vi "HEWH RLT Release Notifier References.vi"(8 "error in (no error)":errorcluster) -> (0 "error out":errorcluster)   [LabVIEW 2020]
uses:
  Type Definitions/HEWH Power Elements.ctl
  Utility/Type Definitions/UTILITY Notifier.ctl
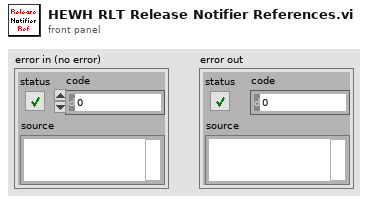
[diagram p1: front panel]
types:
  T1 = typedef "UTILITY Notifier.ctl" = enum16{"Set", "Read", "Release Ref"}
  T2 = typedef "HEWH Power Elements.ctl" = cluster{"UE":bool, "LE":bool, "COMP":bool, "FANS":bool}
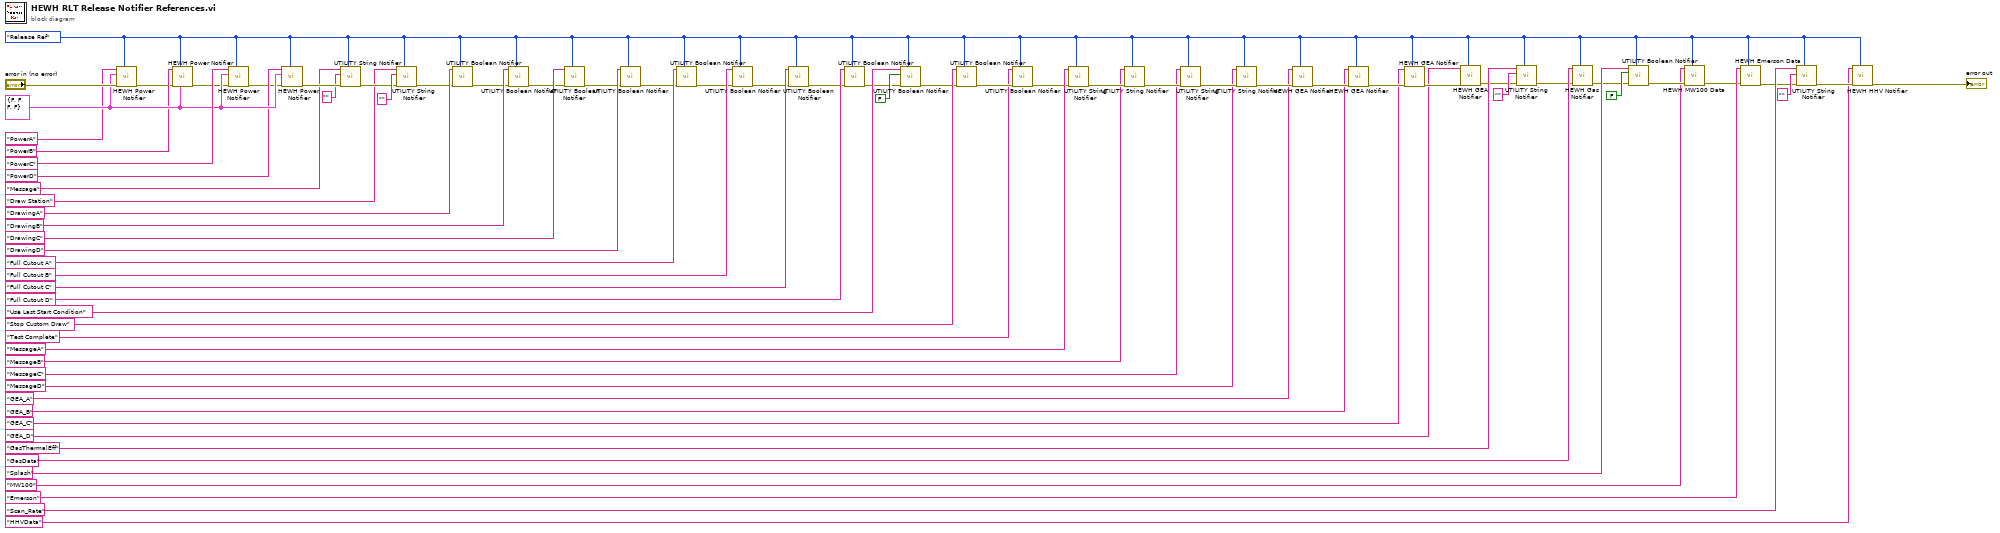
[diagram p0: block diagram]
diagram:
  w2 = UTILITY_Notifier."Release Ref" ("Status")
  w64 = T2 {"UE"=FALSE, "LE"=FALSE, "COMP"=FALSE, "FANS"=FALSE} ("Power Elements")
  n1 = call "HEWH Power Notifier.vi"("Status"=w2, "error in (no error)"="error in (no error)", "Set Status"=w64, "name (unnamed)"="PowerA") -> ("error out"=w59:errorcluster)  [unwired: 6 in, 1 out]
  n2 = call "HEWH Power Notifier.vi"("Status"=w2, "error in (no error)"=w59, "Set Status"=w64, "name (unnamed)"="PowerB") -> ("error out"=w61:errorcluster)  [unwired: 6 in, 1 out]
  n3 = call "HEWH Power Notifier.vi"("Status"=w2, "error in (no error)"=w61, "Set Status"=w64, "name (unnamed)"="PowerC") -> ("error out"=w62:errorcluster)  [unwired: 6 in, 1 out]
  n4 = call "HEWH Power Notifier.vi"("Status"=w2, "error in (no error)"=w62, "Set Status"=w64, "name (unnamed)"="PowerD") -> ("error out"=w69:errorcluster)  [unwired: 6 in, 1 out]
  n5 = call "UTILITY String Notifier.vi"("Status"=w2, "error in (no error)"=w69, "Set Status"="", "name (unnamed)"="Message") -> ("error out"=w71:errorcluster)  [unwired: 6 in, 1 out]
  n6 = call "UTILITY String Notifier.vi"("Status"=w2, "error in (no error)"=w71, "Set Status"="", "name (unnamed)"="Draw Station") -> ("error out"=w53:errorcluster)  [unwired: 6 in, 1 out]
  n7 = call "UTILITY Boolean Notifier.vi"("Status"=w2, "error in (no error)"=w53, "name (unnamed)"="DrawingA") -> ("error out"=w52:errorcluster)  [unwired: 7 in, 1 out]
  n8 = call "UTILITY Boolean Notifier.vi"("Status"=w2, "error in (no error)"=w52, "name (unnamed)"="DrawingB") -> ("error out"=w51:errorcluster)  [unwired: 7 in, 1 out]
  n9 = call "UTILITY Boolean Notifier.vi"("Status"=w2, "error in (no error)"=w51, "name (unnamed)"="DrawingC") -> ("error out"=w50:errorcluster)  [unwired: 7 in, 1 out]
  n10 = call "UTILITY Boolean Notifier.vi"("Status"=w2, "error in (no error)"=w50, "name (unnamed)"="DrawingD") -> ("error out"=w45:errorcluster)  [unwired: 7 in, 1 out]
  n11 = call "UTILITY Boolean Notifier.vi"("Status"=w2, "error in (no error)"=w45, "name (unnamed)"="Full Cutout A") -> ("error out"=w44:errorcluster)  [unwired: 7 in, 1 out]
  n12 = call "UTILITY Boolean Notifier.vi"("Status"=w2, "error in (no error)"=w44, "name (unnamed)"="Full Cutout B") -> ("error out"=w43:errorcluster)  [unwired: 7 in, 1 out]
  n13 = call "UTILITY Boolean Notifier.vi"("Status"=w2, "error in (no error)"=w43, "name (unnamed)"="Full Cutout C") -> ("error out"=w42:errorcluster)  [unwired: 7 in, 1 out]
  n14 = call "UTILITY Boolean Notifier.vi"("Status"=w2, "error in (no error)"=w42, "name (unnamed)"="Full Cutout D") -> ("error out"=w39:errorcluster)  [unwired: 7 in, 1 out]
  n15 = call "UTILITY Boolean Notifier.vi"("Status"=w2, "error in (no error)"=w39, "Set Status"=FALSE, "name (unnamed)"="Use Last Start Condition") -> ("error out"=w38:errorcluster)  [unwired: 6 in, 1 out]
  n16 = call "UTILITY Boolean Notifier.vi"("Status"=w2, "error in (no error)"=w38, "name (unnamed)"="Stop Custom Draw") -> ("error out"=w37:errorcluster)  [unwired: 7 in, 1 out]
  n17 = call "UTILITY Boolean Notifier.vi"("Status"=w2, "error in (no error)"=w37, "name (unnamed)"="Test Complete") -> ("error out"=w34:errorcluster)  [unwired: 7 in, 1 out]
  n18 = call "UTILITY String Notifier.vi"("Status"=w2, "error in (no error)"=w34, "name (unnamed)"="MessageA") -> ("error out"=w31:errorcluster)  [unwired: 7 in, 1 out]
  n19 = call "UTILITY String Notifier.vi"("Status"=w2, "error in (no error)"=w31, "name (unnamed)"="MessageB") -> ("error out"=w32:errorcluster)  [unwired: 7 in, 1 out]
  n20 = call "UTILITY String Notifier.vi"("Status"=w2, "error in (no error)"=w32, "name (unnamed)"="MessageC") -> ("error out"=w33:errorcluster)  [unwired: 7 in, 1 out]
  n21 = call "UTILITY String Notifier.vi"("Status"=w2, "error in (no error)"=w33, "name (unnamed)"="MessageD") -> ("error out"=w27:errorcluster)  [unwired: 7 in, 1 out]
  n22 = call "HEWH GEA Notifier.vi"("Status"=w2, "error in (no error)"=w27, "name (unnamed)"="GEA_A") -> ("error out"=w26:errorcluster)  [unwired: 7 in, 1 out]
  n23 = call "HEWH GEA Notifier.vi"("Status"=w2, "error in (no error)"=w26, "name (unnamed)"="GEA_B") -> ("error out"=w25:errorcluster)  [unwired: 7 in, 1 out]
  n24 = call "HEWH GEA Notifier.vi"("Status"=w2, "error in (no error)"=w25, "name (unnamed)"="GEA_C") -> ("error out"=w24:errorcluster)  [unwired: 7 in, 1 out]
  n25 = call "HEWH GEA Notifier.vi"("Status"=w2, "error in (no error)"=w24, "name (unnamed)"="GEA_D") -> ("error out"=w16:errorcluster)  [unwired: 7 in, 1 out]
  n26 = call "UTILITY String Notifier.vi"("Status"=w2, "error in (no error)"=w16, "Set Status"="", "name (unnamed)"="GasThermalEff") -> ("error out"=w15:errorcluster)  [unwired: 6 in, 1 out]
  n27 = call "HEWH Gas Notifier.vi"("Status"=w2, "error in (no error)"=w15, "name (unnamed)"="GasData") -> ("error out"=w8:errorcluster)  [unwired: 7 in, 1 out]
  n28 = call "UTILITY Boolean Notifier.vi"("Status"=w2, "error in (no error)"=w8, "Set Status"=FALSE, "name (unnamed)"="Splash") -> ("error out"=w12:errorcluster)  [unwired: 6 in, 1 out]
  n29 = call "HEWH MW100 Data.vi"("Status"=w2, "error in (no error)"=w12, "name (unnamed)"="MW100") -> ("error out"=w13:errorcluster)  [unwired: 7 in, 1 out]
  n30 = call "HEWH Emerson Data.vi"("Status"=w2, "error in (no error)"=w13, "name (unnamed)"="Emerson") -> ("error out"=w3:errorcluster)  [unwired: 7 in, 1 out]
  n31 = call "UTILITY String Notifier.vi"("Status"=w2, "error in (no error)"=w3, "Set Status"="", "name (unnamed)"="Scan_Rate") -> ("error out"=w7:errorcluster)  [unwired: 6 in, 1 out]
  n32 = call "HEWH HHV Notifier.vi"("Status"=w2, "error in (no error)"=w7, "name (unnamed)"="HHVData") -> ("error out"=→"error out":errorcluster)  [unwired: 7 in, 1 out]
